vi "sm.main-reverse-delay.vi"   [LabVIEW 2019]
uses:
  <vilib>/rvi/Emulation/niFpgaEmulationIsFPGAContextNoSignature.vi
  <vilib>/rvi/DataTransferAndStorage/Container/Common/niFpgaContainerGetUniqueNameForEmu.vi
  <vilib>/rvi/Memory/Memory_Emulation/niFpgaMemoryEmulationCacheClearOnFirstRun.vi
  <vilib>/rvi/Memory/Memory_Emulation/nirvimemoryEmulationManagerCache_MakeExclusive.vi
  <vilib>/rvi/Memory/Memory_Emulation/niFpgaMemoryEmulationValidateCache.vi
  <vilib>/rvi/Memory/Memory_Emulation/nirvimemoryEmulationManagerCache_InsertValue.vi
  <vilib>/Utility/error.llb/Clear Errors.vi
  <vilib>/rvi/Memory/Memory_Emulation/nirvimemoryEmulationManagerCache_ReleaseExclusive.vi
  <vilib>/rvi/Memory/Memory_Emulation/nirvimemoryEmulationManagerCache_GetValue.vi
  <vilib>/rvi/Memory/Memory_Emulation/nirvimemoryEmulationManagerCache_SetValue.vi
  <vilib>/rvi/Emulation/niFpgaProcessEmulError.vi
  <vilib>/rvi/Emulation/niFpgaSctlEmulationGetInTimedLoop.vi
  rti.global.vi
  <vilib>/rvi/DataTransferAndStorage/Container/XNode/niFpgaContainer.xnode
  <vilib>/rvi/DataTransferAndStorage/Register/Emulation/niFpgaRegisterEmulation.vi
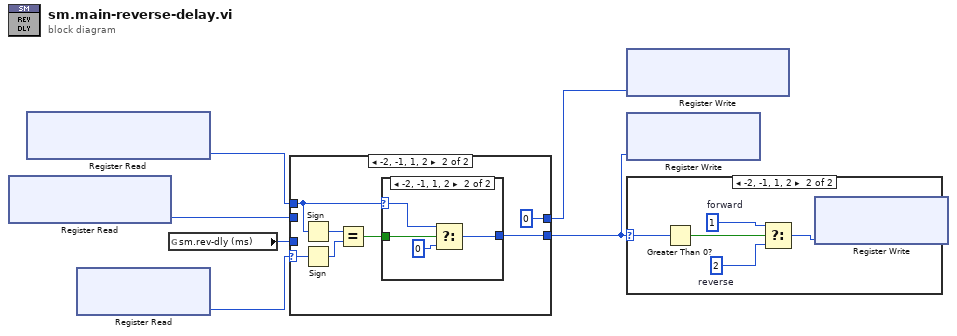
[diagram p0: block diagram]
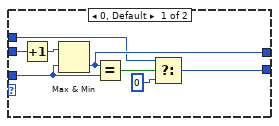
[diagram p3: hidden frame]
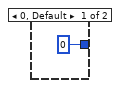
[diagram p4: hidden frame]
diagram:
  n1 = xnode "Register Read"() -> ("Data"=w4:u32)  [unwired: 1 in, 1 out]
  n2 = xnode "Register Read"() -> ("Data"=w3:i8)  [unwired: 1 in, 1 out]
  n3 = xnode "Register Read"() -> ("Data"=w5:i8)  [unwired: 1 in, 1 out]
  n4 = global read "rti.global.vi" "sm.rev-dly (ms)"() -> (w2:u32)
  n5 = case shown="-2, -1, 1, 2" w5 {
    selector: w5 -> [_ w19]
    tunnel: w3 -> [w10 w20]
    tunnel: [w8 w21] -> w1
    tunnel: [w12 u32 0] -> w6
    tunnel: w4 -> [w14 _]
    tunnel: w2 -> [w7 _]
    frame 0, Default {
      n6 = Increment(x=w14) -> (x+1=w13:u32)
      n7 = Max & Min(x=w13, y=w7) -> (min(x,y)=w12:u32)  [unwired: 1 out]
      n8 = Equal?(x=w12, y=w7) -> (x = y?=w11:bool)
      n9 = Select(t=w10, s=w11, f=i8 0) -> (s? t:f=w8:i8)
    }
    frame -2, -1, 1, 2 {
      n10 = Sign(1:w20) -> (0:w18:i8)
      n11 = Sign(1:w19) -> (0:w17:i8)
      n12 = Equal?(x=w18, y=w17) -> (x = y?=w16:bool)
      n13 = case shown="-2, -1, 1, 2" w20 {
        selector: w20 -> [_ w25]
        tunnel: [i8 0 ("Data") w23] -> w21
        tunnel: w16 -> [_ w26]
        frame 0, Default {
        }
        frame -2, -1, 1, 2 {
          n14 = Select(t=w25, s=w26, f=i8 0) -> (s? t:f=w23:i8)
        }
      }
    }
  }
  n15 = xnode "Register Write"("Data"=w6) -> ()  [unwired: 1 in, 1 out]
  n16 = xnode "Register Write"("Data"=w1) -> ()  [unwired: 1 in, 1 out]
  n17 = case shown="-2, -1, 1, 2" w1 {
    selector: w1 -> [_ w31]
    frame 0, Default {
    }
    frame -2, -1, 1, 2 {
      w27 = u8 2  # reverse
      w29 = u8 1  # forward
      n18 = Greater Than 0?(x=w31) -> (x > 0?=w30:bool)
      n19 = Select(t=w29, s=w30, f=w27) -> (s? t:f=w28:u8)
      n20 = xnode "Register Write"("Data"=w28) -> ()  [unwired: 1 in, 1 out]
    }
  }
